vi "Accept.vi"(8 "Error in (no error)":errorcluster, 10 "Log in":T1 {"Priority" items=["EMERGENCY", "ALERT", "CRITICAL", "ERROR", "WARNING", "NOTICE", "INFO", "DEBUG"]}, 11 "LogFilterPriority in":refnum<class "LogFilterPriority.lvclass">) -> (0 "Error out":errorcluster, 2 "Accept":bool, 3 "LogFilterPriority out":refnum<class "LogFilterPriority.lvclass">)   [LabVIEW 2011, in "LogFilterPriority.lvclass"]
uses:
  LogFilterPriority.lvclass
  Log/LogCluster.ctl
  Log/PrioritiesRing.ctl
  LogFilterPriority.lvclass/LogFilterPriority.ctl
  Log/Log.lvclass
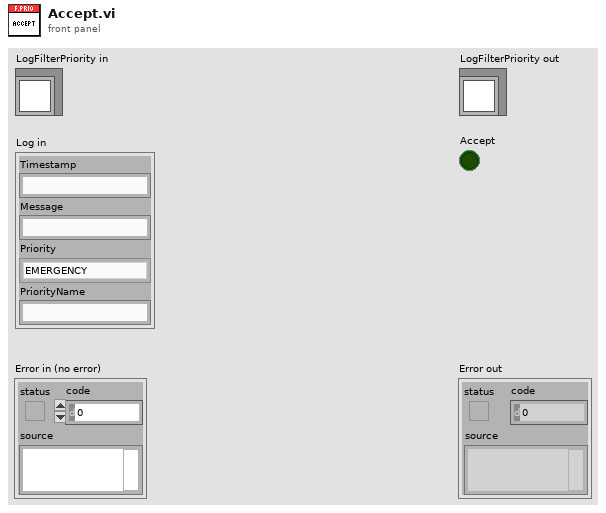
[diagram p1: front panel]
types:
  T1 = typedef "Log.lvclass/LogCluster.ctl" = cluster{"Timestamp":string, "Message":string, "Priority":T2, "PriorityName":string}
  T2 = typedef "Log.lvclass/PrioritiesRing.ctl" = u32
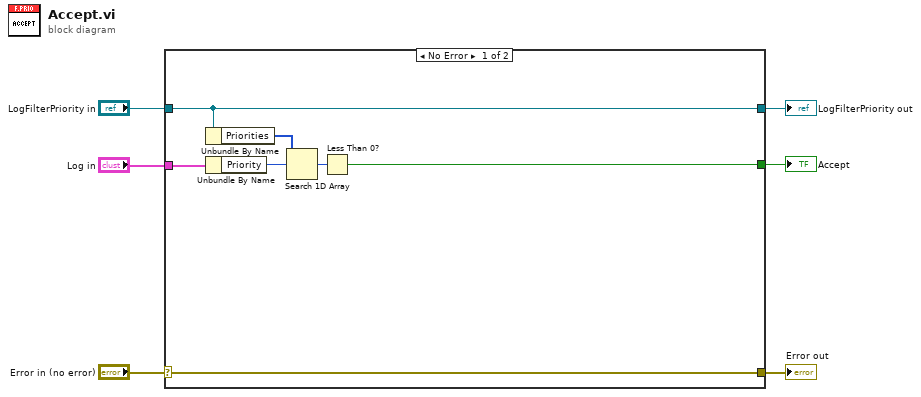
[diagram p0: block diagram]
diagram:
  n1 = case shown="No Error" "Error in (no error)" {
    selector: "Error in (no error)" -> [w13 w15]
    tunnel: [w13 w15] -> w5
    tunnel: [w11 w14] -> w3
    tunnel: "LogFilterPriority in" -> [w11 w14]
    tunnel: "Log in" -> [w12 _]
    tunnel: [w7 _] -> w1
    frame No Error {
      n2 = Unbundle By Name(w11) -> ("Priorities"=w10:T2[])
      n3 = Unbundle By Name(w12) -> ("Priority"=w9:T2)
      n4 = Search 1D Array(1D array=w10, element=w9) -> (index of element=w8:i32)  [unwired: 1 in]
      n5 = Less Than 0?(x=w8) -> (x < 0?=w7:bool)
    }
    frame Error {
    }
  }
  "Error out" <- w5
  "LogFilterPriority out" <- w3
  "Accept" <- w1
